vi "Packet1+Packet2Tx.vi"() -> ()   [LabVIEW 2012]
uses:
  <vilib>/addons/Modulation/Digital/General/MT Generate PSK System Parameters(M).vi
  <instrlib>/niUSRP/niUSRP Write Tx Data (CDB Cluster).vi
  <vilib>/addons/Modulation/niDMT.lvlib
panel:
  in  "Stop the \nTransmission":bool
  out "millisecond timer value 3":u32
  out "Numeric":u32
  out "output cluster":T1
  in  "Referance Cluster":T1={"Tx IQ Sampling\nRate [s/sec]"=500000.0, "Tx Frequency [Hz]"=2500000000.0, "Tx Gain [dB]"=0.0, "Tx Antenna"="TX1"} {"Tx Gain [dB]" format="%#.6p"; "Tx Frequency [Hz]" format="%#.6p"; "Tx IQ Sampling\nRate [s/sec]" format="%#.6p"}
  out "?":dbl
  out "M-PSK (4)":i32
  out "Transmission\n       Stop":bool
  in  "end of data?":bool
  out "Constellation Graph 2":T2(graph) caption="Constellation Graph"
  in  "autoscale 2":bool caption="autoscale"
  out "error out 3":errorcluster
  in  "Tab Control 2":T3(tab)
  in  "Enter Information":string
  in  "Packet Parameters 2":T4={"Guard Bits "=30, "Sync Bits"=20, "Message Bits"=128}
  in  "Packet Pad \n[samples] 2":i32=200
  in  "Blank Frame \n[samples] 2":i32=500
  out "Number of Packets in Message 2":i32=46
  in  "PN sequence order\nfor Sync Bits 2":i32=31 caption="PN sequence order (9)"
  in  "Packet Repeat 2":i32=2
  in  "Pulse Shaping Filter Parameters 2":T5={"Alpha"=0.5, "Filter Length"=6, "TX Filter"=enum."Root Raised Cos"} caption="Pulse Shaping Filter" {"Alpha" format="%.2f"}
  out "Actual Tx Parameters 2":T1={"Tx IQ Sampling\nRate [s/sec]"=200000.0, "Tx Frequency [Hz]"=2500000000.0, "Tx Gain [dB]"=0.0, "Tx Antenna"="TX1"} {"Tx Gain [dB]" format="%#.6p"; "Tx Frequency [Hz]" format="%#.6p"; "Tx IQ Sampling\nRate [s/sec]" format="%#.6p"}
  out "error out 2":errorcluster
  in  "Queue Length 2":i32=10
  in  "BPSK System Parameters 9":T6={"Samples per Symbol"=8, "symbol map"=[], "Differential PSK"=enum."disable", "PSK type"=0} caption="BPSK System Parameters" {"PSK type" items=["normal", "shifted", "offset"]; "symbol map" format="%.3f"}
  in  "BPSK System Parameters 8":T6={"Samples per Symbol"=8, "symbol map"=[], "Differential PSK"=enum."disable", "PSK type"=0} caption="BPSK System Parameters" {"PSK type" items=["normal", "shifted", "offset"]; "symbol map" format="%.3f"}
  in  "BPSK System Parameters 7":T6={"Samples per Symbol"=8, "symbol map"=[], "Differential PSK"=enum."disable", "PSK type"=0} caption="BPSK System Parameters" {"PSK type" items=["normal", "shifted", "offset"]; "symbol map" format="%.3f"}
  in  "BPSK System Parameters 6":T6={"Samples per Symbol"=8, "symbol map"=[], "Differential PSK"=enum."disable", "PSK type"=0} caption="BPSK System Parameters" {"PSK type" items=["normal", "shifted", "offset"]; "symbol map" format="%.3f"}
  in  "BPSK System Parameters 5":T6={"Samples per Symbol"=8, "symbol map"=[], "Differential PSK"=enum."disable", "PSK type"=0} caption="BPSK System Parameters" {"PSK type" items=["normal", "shifted", "offset"]; "symbol map" format="%.3f"}
  in  "BPSK System Parameters 4":T6={"Samples per Symbol"=8, "symbol map"=[], "Differential PSK"=enum."disable", "PSK type"=0} caption="BPSK System Parameters" {"PSK type" items=["normal", "shifted", "offset"]; "symbol map" format="%.3f"}
  in  "BPSK System Parameters 3":T6={"Samples per Symbol"=8, "symbol map"=[], "Differential PSK"=enum."disable", "PSK type"=0} caption="BPSK System Parameters" {"PSK type" items=["normal", "shifted", "offset"]; "symbol map" format="%.3f"}
  out "Symbol Rate\n[symbols/sec] 2":dbl=25000.0 format="%#.6p"
  out "millisecond timer value":u32
  in  "Stop after \nControl Signal Reached":bool
  in  "Tab Control":T3(tab)
  in  "Enter Control Signal\n1,2 or 3":string="Two roads diverged in a yellow wood,\nAnd sorry I could not travel both\nAnd be one traveler, long I stood\nAnd looked down one as far as I could\nTo where it bent in the undergrowth.\n\nThen took the other, as just as fair,\nAnd having perhaps the better claim,\nBecause it was grassy and wanted wear;\nThough as for that the passing there\nHad worn them really about the same.\n\nAnd both that morning equally lay\nIn leaves no step had trodden black.\nOh, I kept the first for another day!\nYet knowing how way leads on to way,\nI doubted if I should ever come back.\n\nI shall be telling this with a sigh\nSomewhere ages and ages hence:\nTwo roads diverged in a wood, and I--\nI took the one less traveled by,\nAnd that has made all the difference.\n"
  in  "Packet Parameters":T4={"Guard Bits "=30, "Sync Bits"=20, "Message Bits"=128}
  in  "Packet Pad \n[samples]":i32=200
  in  "Blank Frame \n[samples]":i32=500
  out "Number of Packets in Message":i32=46
  in  "PN sequence order\nfor Sync Bits":i32=31 caption="PN sequence order (9)"
  in  "Packet Repeat":i32=2
  in  "Select PSK Modulation Format":T7(tab)=enum."QPSK" caption="PSK"
  in  "BPSK System Parameters":T6={"Samples per Symbol"=8, "symbol map"=[], "Differential PSK"=enum."disable", "PSK type"=0} {"PSK type" items=["normal", "shifted", "offset"]; "symbol map" format="%.3f"}
  in  "QPSK System Parameters":T6={"Samples per Symbol"=8, "symbol map"=[], "Differential PSK"=enum."disable", "PSK type"=0} {"PSK type" items=["normal", "shifted", "offset"]; "symbol map" format="%.3f"}
  in  "pi/4 DQPSK System Parameters":T6={"Samples per Symbol"=8, "symbol map"=[], "Differential PSK"=enum."enable", "PSK type"=1} {"PSK type" items=["normal", "shifted", "offset"]; "symbol map" format="%.3f"}
  in  "OQPSK System Parameters":T6={"Samples per Symbol"=8, "symbol map"=[], "Differential PSK"=enum."disable", "PSK type"=2} {"PSK type" items=["normal", "shifted", "offset"]; "symbol map" format="%.3f"}
  in  "8-PSK System Parameters":T6={"Samples per Symbol"=8, "symbol map"=[], "Differential PSK"=enum."disable", "PSK type"=0} {"PSK type" items=["normal", "shifted", "offset"]; "symbol map" format="%.3f"}
  in  "16-PSK System Parameters":T6={"Samples per Symbol"=8, "symbol map"=[], "Differential PSK"=enum."disable", "PSK type"=0} {"PSK type" items=["normal", "shifted", "offset"]; "symbol map" format="%.3f"}
  in  "M":i32=4 min=2 step=2
  in  "Custom System Parameters":T6={"Samples per Symbol"=8, "symbol map"=[], "Differential PSK"=enum."disable", "PSK type"=0} {"PSK type" items=["normal", "shifted", "offset"]; "symbol map" format="%.3f"}
  in  "Pulse Shaping Filter Parameters":T5={"Alpha"=0.5, "Filter Length"=6, "TX Filter"=enum."Root Raised Cos"} caption="Pulse Shaping Filter" {"Alpha" format="%.2f"}
  in  "Tx Parameters":T1={"Tx IQ Sampling\nRate [s/sec]"=500000.0, "Tx Frequency [Hz]"=2500000000.0, "Tx Gain [dB]"=0.0, "Tx Antenna"="TX1"} {"Tx Gain [dB]" format="%#.6p"; "Tx Frequency [Hz]" format="%#.6p"; "Tx IQ Sampling\nRate [s/sec]" format="%#.6p"}
  out "Actual Tx Parameters":T1={"Tx IQ Sampling\nRate [s/sec]"=200000.0, "Tx Frequency [Hz]"=2500000000.0, "Tx Gain [dB]"=0.0, "Tx Antenna"="TX1"} {"Tx Gain [dB]" format="%#.6p"; "Tx Frequency [Hz]" format="%#.6p"; "Tx IQ Sampling\nRate [s/sec]" format="%#.6p"}
  in  "USRP IP address":refnum<k15>="192.168.10.2"
  out "error out":errorcluster
  in  "Queue Length":i32=10
  out "Constellation Graph":T2(graph)
  in  "autoscale":bool
  out "Symbol Rate\n[symbols/sec]":dbl=25000.0 format="%#.6p"
  in  "stop":bool
  # "Guard\nBand"
  # "Sync\nSeq"
  # "Packet\nNumber"
  # "Pad\nData"
  # "Blank\nFrame"
  # "Data"
  # "Guard\nBand"
  # "Sync\nSeq"
  # "Packet\nNumber"
  # "Pad\nData"
  # "Blank\nFrame"
  # "Data"
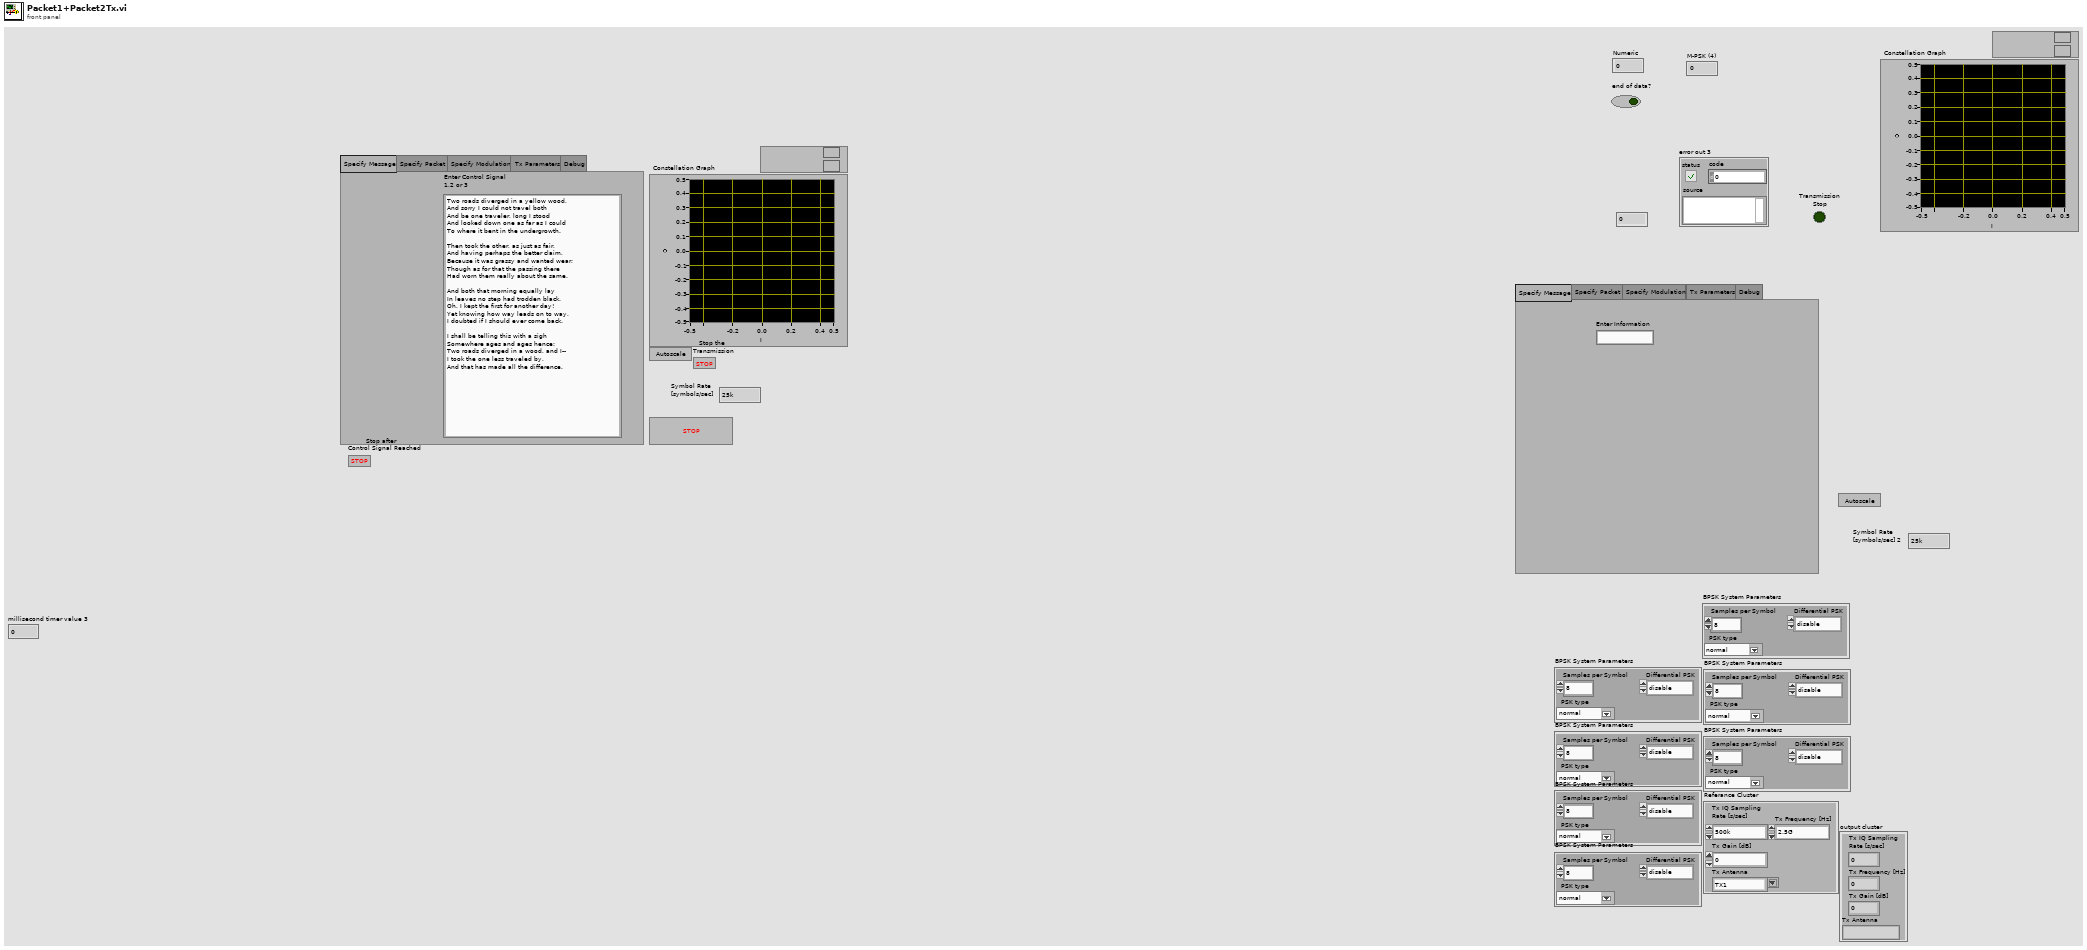
[diagram p1: front panel]
types:
  T1 = cluster{"Tx IQ Sampling\nRate [s/sec]":dbl, "Tx Frequency [Hz]":dbl, "Tx Gain [dB]":dbl, "Tx Antenna":string}
  T2 = cluster{"Decimated Array":dbl[], "Decimated Array":dbl[]}[]
  T3 = enum32{"Specify Message", "Specify Packet", "Specify Modulation", "Tx Parameters", "Debug"}
  T4 = cluster{"Guard Bits ":i32, "Sync Bits":i32, "Message Bits":i32}
  T5 = cluster{"Alpha":dbl, "Filter Length":i32, "TX Filter":enum16{"none", "Raised Cosine", "Root Raised Cos", "Gaussian"}}
  T6 = cluster{"Samples per Symbol":i32, "symbol map":cdb[], "Differential PSK":enum16{"disable", "enable"}, "PSK type":u16}
  T7 = enum32{"BPSK", "QPSK", "pi/4DQPSK", "OQPSK", "8-PSK", "16-PSK", "Custom"}
  T8 = cluster{"samples per symbol (16)":i32, "symbol map":cdb[], "differential PSK":enum16{"disable", "enable"}, "PSK type":u16}
  T9 = cluster{"s? t:f":cluster{"t0":dbl, "dt":dbl, "Y":cdb[]}, i32}
  T10 = cluster{"output complex waveform":cluster{"t0":dbl, "dt":dbl, "Y":cdb[]}, i32}
  T11 = cluster{"constellation":dbl[], "oversampled data":dbl[]}[]
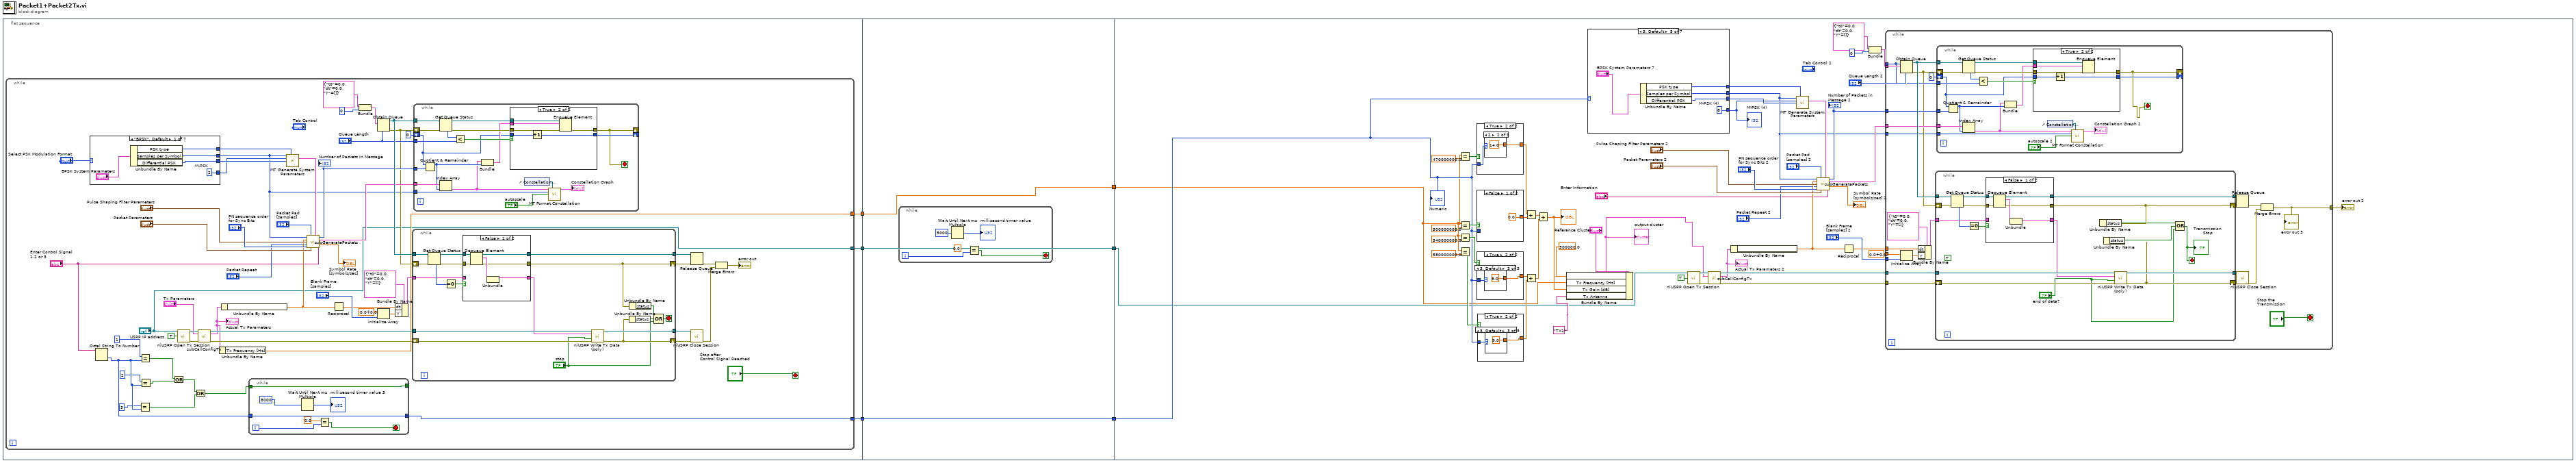
[diagram p0: block diagram]
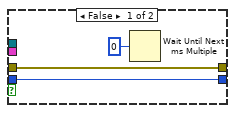
[diagram p2: hidden frame]
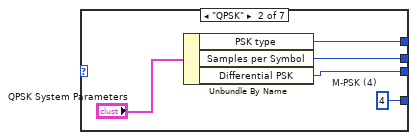
[diagram p3: hidden frame]
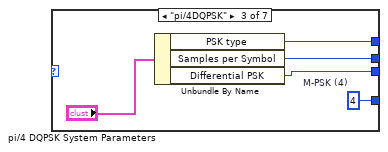
[diagram p4: hidden frame]
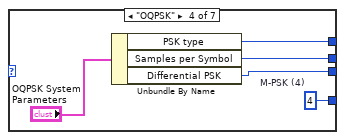
[diagram p5: hidden frame]
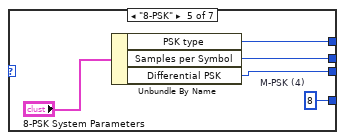
[diagram p6: hidden frame]
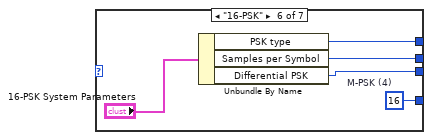
[diagram p7: hidden frame]
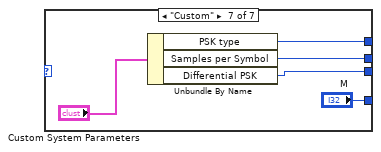
[diagram p8: hidden frame]
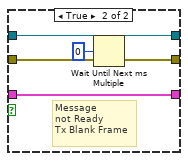
[diagram p9: hidden frame]
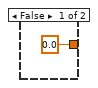
[diagram p10: hidden frame]
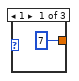
[diagram p11: hidden frame]
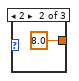
[diagram p12: hidden frame]
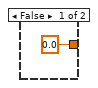
[diagram p13: hidden frame]
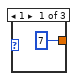
[diagram p14: hidden frame]
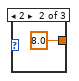
[diagram p15: hidden frame]
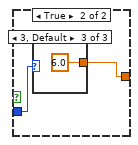
[diagram p16: hidden frame]
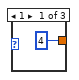
[diagram p17: hidden frame]
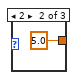
[diagram p18: hidden frame]
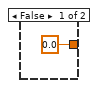
[diagram p19: hidden frame]
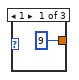
[diagram p20: hidden frame]
diagram:
  n1 = flat-sequence {
    tunnel: [w9] -> w5
    tunnel: [w8] -> w3
    tunnel: [w7] -> w1
    tunnel: [w166] -> w6
    tunnel: w5 -> [w166]
    tunnel: [w165] -> w4
    tunnel: w3 -> [w165]
    tunnel: [w164] -> w2
    tunnel: w1 -> [w164]
    tunnel: w6 -> [w174]
    tunnel: w4 -> [w173]
    tunnel: w2 -> [w172]
    frame #0 {
      n2 = while {
        tunnel: [w13] -> w9
        tunnel: [w11] -> w8
        tunnel: ["USRP IP address"] -> w7
        stop <- "Stop after \nControl Signal Reached" stop-if-true
        n3 = case shown="\"BPSK\", Default" "Select PSK Modulation Format" {
          tunnel: [w102 w106 w114 w119 w124 w130 w133] -> w27
          tunnel: [w103 w108 w113 w118 w123 w129 w134] -> w64
          tunnel: [w105 w110 w115 w120 w122 w128 "M"] -> w46
          tunnel: [w104 w109 w112 w117 w125 w127 w135] -> w35
          frame "BPSK", Default {
            w105 = 2  # M-PSK
            n4 = Unbundle By Name("BPSK System Parameters") -> ("PSK type"=w104:u16, "Samples per Symbol"=w102:i32, "Differential PSK"=w103:enum16{"disable", "enable"})
          }
          frame "QPSK" {
            w110 = 4  # M-PSK (4)
            n5 = Unbundle By Name("QPSK System Parameters") -> ("PSK type"=w109:u16, "Samples per Symbol"=w106:i32, "Differential PSK"=w108:enum16{"disable", "enable"})
          }
          frame "pi/4DQPSK" {
            w115 = 4  # M-PSK (4)
            n6 = Unbundle By Name("pi/4 DQPSK System Parameters") -> ("PSK type"=w112:u16, "Samples per Symbol"=w114:i32, "Differential PSK"=w113:enum16{"disable", "enable"})
          }
          frame "OQPSK" {
            w120 = 4  # M-PSK (4)
            n7 = Unbundle By Name("OQPSK System Parameters") -> ("PSK type"=w117:u16, "Samples per Symbol"=w119:i32, "Differential PSK"=w118:enum16{"disable", "enable"})
          }
          frame "8-PSK" {
            w122 = 8  # M-PSK (4)
            n8 = Unbundle By Name("8-PSK System Parameters") -> ("PSK type"=w125:u16, "Samples per Symbol"=w124:i32, "Differential PSK"=w123:enum16{"disable", "enable"})
          }
          frame "16-PSK" {
            w128 = 16  # M-PSK (4)
            n9 = Unbundle By Name("16-PSK System Parameters") -> ("PSK type"=w127:u16, "Samples per Symbol"=w130:i32, "Differential PSK"=w129:enum16{"disable", "enable"})
          }
          frame "Custom" {
            n10 = Unbundle By Name("Custom System Parameters") -> ("PSK type"=w135:u16, "Samples per Symbol"=w133:i32, "Differential PSK"=w134:enum16{"disable", "enable"})
          }
        }
        n11 = Octal String To Number(4:"Enter Control Signal\n1,2 or 3") -> (0:w18:u32)  [unwired: 2 in, 1 out]
        n12 = Equal?(x=3, y=w18) -> (x = y?=w20:bool)
        n13 = Equal?(x=1, y=w18) -> (x = y?=w23:bool)
        n14 = Equal?(x=2, y=w18) -> (x = y?=w22:bool)
        n15 = Or(x=w23, y=w22) -> (x .or. y?=w21:bool)
        n16 = call <instrlib>:"niUSRP Open Tx Session.vi"("device names"="USRP IP address", "reset"=TRUE) -> ("session handle out"=w38:refnum<k15>, "error out"=w37:errorcluster)  [unwired: 12 in]
        n17 = Or(x=w21, y=w20) -> (x .or. y?=w19:bool)
        n18 = call "subCallConfigTx.vi"("session handle"=w38, "Tx Parameters"="Tx Parameters", "error in"=w37) -> ("session handle out"=w45:refnum<k15>, "Actual Tx Parameters"=w12:T1, "error out"=w50:errorcluster)  [unwired: 10 in]
        "Actual Tx Parameters" <- w12
        n19 = Unbundle By Name(w12) -> ("Tx Frequency [Hz]"=w11:dbl)
        n20 = Unbundle By Name(w12) -> ("Tx IQ Sampling\nRate [s/sec]"=w28:dbl)
        n21 = while {
          tunnel: w19 -> [w71]
          tunnel: [w71] -> _
          tunnel: w18 -> [w70]
          tunnel: [w70] -> w13
          i -> [w68]
          stop <- w67 stop-if-true
          n22 = Wait Until Next ms Multiple(millisecond multiple=u32 8000) -> (millisecond timer value=→"millisecond timer value 3":u32)
          n23 = Equal?(x=0.0, y=w68) -> (x = y?=w67:bool)
        }
        n24 = call-poly <vilib>:"MT Generate System Parameters.vi"("samples per symbol (16)"=w27, "PSK type"=w35, "M-PSK (4)"=w46, "differential PSK"=w64) -> ("PSK system parameters"=w36:T8)  [unwired: 9 in, 2 out]
        n25 = call "subGeneratePackets.vi"("Samples per Symbol"=w27, "Packet Pad \n[samples]"="Packet Pad \n[samples]", "PSK system parameters"=w36, "Tx IQ Sampling\nRate [s/sec]"=w28, "Pulse Shaping Filter Parameters"="Pulse Shaping Filter Parameters", "Packet Repeat"="Packet Repeat", "PN sequence order\nfor Sync Bits"="PN sequence order\nfor Sync Bits", "Packet Parameters"="Packet Parameters", "Message Text"="Enter Control Signal\n1,2 or 3") -> ("Number of Packets"=w44:i32, "Packets"=w52:cluster{"t0":dbl, "dt":dbl, "Y":cdb[]}[], "Symbol Rate"=→"Symbol Rate\n[symbols/sec]":dbl)  [unwired: 4 in]
        "Number of Packets in Message" <- w44
        n26 = Reciprocal(x=w28) -> (1/x=w47:dbl)
        n27 = Bundle("s? t:f"=cluster{"t0":dbl, "dt":dbl, "Y":cdb[]} {"t0"=0.0, "dt"=0.0, "Y"=[]}, 0) -> (w55:T9)  [unwired: 1 in]
        n28 = Obtain Queue(max queue size (-1, unlimited)="Queue Length", element data type=w55) -> (queue out=w61:refnum<queue>, error out=w40:errorcluster)  [unwired: 3 in, 1 out]
        n29 = Initialize Array(cdb 0.0+0.0i ("element"), "Blank Frame \n[samples]") -> (w60:cdb[])
        n30 = Bundle By Name(cluster=cluster{"t0":dbl, "dt":dbl, "Y":cdb[]} {"t0"=0.0, "dt"=0.0, "Y"=[]} ("s? t:f"), "dt"=w47, "Y"=w60) -> (w59:cluster{"t0":dbl, "dt":dbl, "Y":cdb[]})
        n31 = while {
          tunnel: w45 -> [w144]
          shift-right: [w141] -> w49
          shift-left: w50 -> [w145]
          tunnel: w61 -> [w153]
          tunnel: w59 -> [w150]
          tunnel: [w149] -> w58
          tunnel: [w143] -> w48
          shift-right: [w138] -> w57
          shift-left: w40 -> [w146]
          stop <- w140 stop-if-true
          n32 = Get Queue Status(queue=w153, error in (no error)=w146) -> (queue out=w148:refnum<queue>, error out=w147:errorcluster, # elements in queue=w152:i32)  [unwired: 1 in, 5 out]
          n33 = Equal To 0?(x=w152) -> (x = 0?=w151:bool)
          n34 = case shown="False" w151 {
            tunnel: w150 -> [_ w163]
            tunnel: [w155 w163] -> w136
            tunnel: [w159 w161] -> w149
            tunnel: [w154 w162] -> w138
            tunnel: w148 -> [w158 w161]
            tunnel: w147 -> [w157 w162]
            frame False {
              n35 = Dequeue Element(queue=w158, error in (no error)=w157) -> (queue out=w159:refnum<queue>, element=w156:T9, error out=w154:errorcluster)  [unwired: 1 in, 1 out]
              n36 = Unbundle(w156) -> ("s? t:f"=w155:cluster{"t0":dbl, "dt":dbl, "Y":cdb[]})  [unwired: 1 out]
            }
            frame True {
              # "Message\nnot Ready\nTx Blank Frame"
              n37 = Wait Until Next ms Multiple(millisecond multiple=u32 0) -> ()  [unwired: 1 out]
            }
          }
          n38 = call-poly <instrlib>:"niUSRP Write Tx Data (poly).vi"("session handle"=w144, "data"=w136, "end of data?"="stop", "error in (no error)"=w145) -> ("session handle out"=w143:refnum<k15>, "error out"=w141:errorcluster)  [unwired: 10 in]
          n39 = Unbundle By Name(w141) -> ("status"=w142:bool)
          n40 = Unbundle By Name(w138) -> ("status"=w137:bool)
          n41 = Compound Arithmetic op=OR(w137, w142, "stop") -> (w140:bool)
        }
        n42 = while {
          tunnel: w61 -> [w91]
          shift-right: [w84] -> _
          shift-left: 0 -> [w80]
          tunnel: w52 -> [w81]
          tunnel: "Queue Length" -> [w83]
          tunnel: w44 -> [w82]
          shift-right: [w78] -> _
          shift-left: w40 -> [w86]
          tunnel: w27 -> [w75]
          stop <- w78 stop-if-true
          n43 = Quotient & Remainder(x=w80, y=w82) -> (x-y*floor(x/y)=w79:i32)  [unwired: 1 out]
          n44 = Index Array(array=w81, index=w79) -> (element=w73:cluster{"t0":dbl, "dt":dbl, "Y":cdb[]})
          n45 = Get Queue Status(queue=w91, error in (no error)=w86) -> (queue out=w90:refnum<queue>, error out=w87:errorcluster, # elements in queue=w89:i32)  [unwired: 1 in, 5 out]
          n46 = Less?(x=w89, y=w83) -> (x < y?=w88:bool)
          n47 = Bundle("output complex waveform"=w73, w79) -> (w85:T10)  [unwired: 1 in]
          n48 = case shown="True" w88 {
            tunnel: w87 -> [w92 w100]
            tunnel: w90 -> [_ w99]
            tunnel: [w92 w98] -> w78
            tunnel: w85 -> [_ w97]
            tunnel: w80 -> [w94 w96]
            tunnel: [w94 w95] -> w84
            frame False {
              n49 = Wait Until Next ms Multiple(millisecond multiple=u32 0) -> ()  [unwired: 1 out]
            }
            frame True {
              n50 = Increment(x=w96) -> (x+1=w95:i32)
              n51 = Enqueue Element(queue=w99, element=w97, error in (no error)=w100) -> (error out=w98:errorcluster)  [unwired: 1 in, 2 out]
            }
          }
          n52 = control-ref of="Constellation Graph"() -> (w76:refnum<vi>)
          n53 = call <vilib>:"MT Format Constellation.vi"("waveform"=w73, "constellation reference"=w76, "samples per symbol"=w75, "autoscale"="autoscale") -> ("constellation graph"=→"Constellation Graph":T11)  [unwired: 1 in, 10 out]
        }
        n54 = Release Queue(queue=w58, error in (no error)=w57) -> (error out=w34:errorcluster)  [unwired: 3 out]
        n55 = call <instrlib>:"niUSRP Close Session.vi"("session handle"=w48, "error in (no error)"=w49) -> ("error out"=w33:errorcluster)  [unwired: 13 in]
        n56 = Merge Errors(w34, w33) -> (→"error out":errorcluster)
      }
    }
    frame #1 {
      n57 = while {
        i -> [w169]
        stop <- w168 stop-if-true
        n58 = Wait Until Next ms Multiple(millisecond multiple=u32 5000) -> (millisecond timer value=→"millisecond timer value":u32)
        n59 = Equal?(x=0.0, y=w169) -> (x = y?=w168:bool)
      }
    }
    frame #2 {
      n60 = Equal?(x=w173, y=470000000.0) -> (x = y?=w182:bool)
      n61 = Equal?(x=w173, y=500000000.0) -> (x = y?=w183:bool)
      n62 = Equal?(x=w173, y=540000000.0) -> (x = y?=w184:bool)
      n63 = Equal?(x=w173, y=580000000.0) -> (x = y?=w176:bool)
      n64 = case shown="True" w182 {
        tunnel: [0.0 w242] -> w191
        tunnel: w174 -> [_ w243]
        frame False {
        }
        frame True {
          n65 = case shown="2" w243 {
            tunnel: [9 14.0 18.0] -> w242
            frame 1 {
            }
            frame 2 {
            }
            frame 3, Default {
            }
          }
        }
      }
      n66 = case shown="False" w183 {
        tunnel: [0.0 w236] -> w190
        tunnel: w174 -> [_ w237]
        frame False {
        }
        frame True {
          n67 = case shown="3, Default" w237 {
            tunnel: [4 5.0 6.0] -> w236
            frame 1 {
            }
            frame 2 {
            }
            frame 3, Default {
            }
          }
        }
      }
      n68 = case shown="True" w184 {
        tunnel: [0.0 w230] -> w189
        tunnel: w174 -> [_ w231]
        frame False {
        }
        frame True {
          n69 = case shown="3, Default" w231 {
            tunnel: [7 8.0 9.0] -> w230
            frame 1 {
            }
            frame 2 {
            }
            frame 3, Default {
            }
          }
        }
      }
      n70 = case shown="True" w176 {
        tunnel: [0.0 w224] -> w175
        tunnel: w174 -> [_ w225]
        frame False {
        }
        frame True {
          n71 = case shown="3, Default" w225 {
            tunnel: [7 8.0 9.0] -> w224
            frame 1 {
            }
            frame 2 {
            }
            frame 3, Default {
            }
          }
        }
      }
      n72 = Add(x=w191, y=w190) -> (x+y=w193:dbl)
      n73 = Add(x=w189, y=w175) -> (x+y=w192:dbl)
      n74 = Add(x=w193, y=w192) -> (x+y=w180:dbl)
      "?" <- w180
      n75 = Bundle By Name(cluster="Referance Cluster", "Tx IQ Sampling\nRate [s/sec]"=500000.0, "Tx Frequency [Hz]"=w173, "Tx Gain [dB]"=w180, "Tx Antenna"="TX1") -> (w178:T1)
      "output cluster" <- w178
      n76 = case shown="3, Default" w174 {
        tunnel: [w328 w333 w340 w345 w350 w356 w359] -> w197
        tunnel: [w329 w334 w339 w344 w349 w355 w360] -> w222
        tunnel: [w331 w336 w341 w346 w348 w354 0 ("M-PSK (4)")] -> w213
        tunnel: [w330 w335 w338 w343 w351 w353 w361] -> w203
        frame 1 {
          w331 = 2  # M-PSK
          n77 = Unbundle By Name("BPSK System Parameters 3") -> ("PSK type"=w330:u16, "Samples per Symbol"=w328:i32, "Differential PSK"=w329:enum16{"disable", "enable"})
        }
        frame 2 {
          w336 = 4  # M-PSK (4)
          n78 = Unbundle By Name("BPSK System Parameters 4") -> ("PSK type"=w335:u16, "Samples per Symbol"=w333:i32, "Differential PSK"=w334:enum16{"disable", "enable"})
        }
        frame 4 {
          w341 = 4  # M-PSK (4)
          n79 = Unbundle By Name("BPSK System Parameters 5") -> ("PSK type"=w338:u16, "Samples per Symbol"=w340:i32, "Differential PSK"=w339:enum16{"disable", "enable"})
        }
        frame 5 {
          w346 = 4  # M-PSK (4)
          n80 = Unbundle By Name("BPSK System Parameters 6") -> ("PSK type"=w343:u16, "Samples per Symbol"=w345:i32, "Differential PSK"=w344:enum16{"disable", "enable"})
        }
        frame 3, Default {
          w348 = 8  # M-PSK (4)
          n81 = Unbundle By Name("BPSK System Parameters 7") -> ("PSK type"=w351:u16, "Samples per Symbol"=w350:i32, "Differential PSK"=w349:enum16{"disable", "enable"})
        }
        frame 6 {
          w354 = 16  # M-PSK (4)
          n82 = Unbundle By Name("BPSK System Parameters 8") -> ("PSK type"=w353:u16, "Samples per Symbol"=w356:i32, "Differential PSK"=w355:enum16{"disable", "enable"})
        }
        frame 7 {
          n83 = Unbundle By Name("BPSK System Parameters 9") -> ("PSK type"=w361:u16, "Samples per Symbol"=w359:i32, "Differential PSK"=w360:enum16{"disable", "enable"})
        }
      }
      "M-PSK (4)" <- w213
      n84 = call <instrlib>:"niUSRP Open Tx Session.vi"("device names"=w172, "reset"=TRUE) -> ("session handle out"=w206:refnum<k15>, "error out"=w205:errorcluster)  [unwired: 12 in]
      n85 = call "subCallConfigTx.vi"("session handle"=w206, "Tx Parameters"=w178, "error in"=w205) -> ("session handle out"=w212:refnum<k15>, "Actual Tx Parameters"=w211:T1, "error out"=w215:errorcluster)  [unwired: 10 in]
      "Actual Tx Parameters 2" <- w211
      n86 = Unbundle By Name(w211) -> ("Tx IQ Sampling\nRate [s/sec]"=w198:dbl)
      n87 = call-poly <vilib>:"MT Generate System Parameters.vi"("samples per symbol (16)"=w197, "PSK type"=w203, "M-PSK (4)"=w213, "differential PSK"=w222) -> ("PSK system parameters"=w204:T8)  [unwired: 9 in, 2 out]
      n88 = call "subGeneratePackets.vi"("Samples per Symbol"=w197, "Packet Pad \n[samples]"="Packet Pad \n[samples] 2", "PSK system parameters"=w204, "Tx IQ Sampling\nRate [s/sec]"=w198, "Pulse Shaping Filter Parameters"="Pulse Shaping Filter Parameters 2", "Packet Repeat"="Packet Repeat 2", "PN sequence order\nfor Sync Bits"="PN sequence order\nfor Sync Bits 2", "Packet Parameters"="Packet Parameters 2", "Message Text"="Enter Information") -> ("Number of Packets"=w210:i32, "Packets"=w216:cluster{"t0":dbl, "dt":dbl, "Y":cdb[]}[], "Symbol Rate"=→"Symbol Rate\n[symbols/sec] 2":dbl)  [unwired: 4 in]
      "Number of Packets in Message 2" <- w210
      n89 = Reciprocal(x=w198) -> (1/x=w214:dbl)
      n90 = Bundle("s? t:f"=cluster{"t0":dbl, "dt":dbl, "Y":cdb[]} {"t0"=0.0, "dt"=0.0, "Y"=[]}, 0) -> (w218:T9)  [unwired: 1 in]
      n91 = while {
        tunnel: cdb 0.0+0.0i ("element") -> [w270]
        tunnel: "Blank Frame \n[samples] 2" -> [w269]
        tunnel: w218 -> [w263]
        tunnel: "Queue Length 2" -> [w261]
        tunnel: w216 -> [w260]
        tunnel: w215 -> [w259]
        tunnel: w214 -> [w256]
        tunnel: w212 -> [w255]
        tunnel: w210 -> [w254]
        tunnel: [w249] -> w202
        tunnel: w197 -> [w248]
        stop <- "Stop the \nTransmission" stop-if-true
        n92 = Obtain Queue(max queue size (-1, unlimited)=w261, element data type=w263) -> (queue out=w268:refnum<queue>, error out=w252:errorcluster)  [unwired: 3 in, 1 out]
        n93 = Initialize Array(w270, w269) -> (w267:cdb[])
        n94 = Bundle By Name(cluster=cluster{"t0":dbl, "dt":dbl, "Y":cdb[]} {"t0"=0.0, "dt"=0.0, "Y"=[]} ("s? t:f"), "dt"=w256, "Y"=w267) -> (w266:cluster{"t0":dbl, "dt":dbl, "Y":cdb[]})
        n95 = while {
          tunnel: w255 -> [w307]
          shift-right: [w304] -> w258
          shift-left: w259 -> [w308]
          tunnel: w268 -> [w316]
          tunnel: w266 -> [w313]
          tunnel: [w312] -> w265
          tunnel: [w306] -> w257
          shift-right: [w303] -> w264
          shift-left: w252 -> [w309]
          stop <- w300 stop-if-true
          (unwired) TRUE
          n96 = Get Queue Status(queue=w316, error in (no error)=w309) -> (queue out=w311:refnum<queue>, error out=w310:errorcluster, # elements in queue=w315:i32)  [unwired: 1 in, 5 out]
          n97 = Equal To 0?(x=w315) -> (x = 0?=w314:bool)
          n98 = case shown="False" w314 {
            tunnel: w313 -> [_ w326]
            tunnel: [w318 w326] -> w301
            tunnel: [w322 w324] -> w312
            tunnel: [w317 w325] -> w303
            tunnel: w311 -> [w321 w324]
            tunnel: w310 -> [w320 w325]
            frame False {
              n99 = Dequeue Element(queue=w321, error in (no error)=w320) -> (queue out=w322:refnum<queue>, element=w319:T9, error out=w317:errorcluster)  [unwired: 1 in, 1 out]
              n100 = Unbundle(w319) -> ("s? t:f"=w318:cluster{"t0":dbl, "dt":dbl, "Y":cdb[]})  [unwired: 1 out]
            }
            frame True {
              # "Message\nnot Ready\nTx Blank Frame"
              n101 = Wait Until Next ms Multiple(millisecond multiple=u32 0) -> ()  [unwired: 1 out]
            }
          }
          n102 = Unbundle By Name(w303) -> ("status"=w302:bool)
          n103 = call-poly <instrlib>:"niUSRP Write Tx Data (poly).vi"("session handle"=w307, "data"=w301, "end of data?"="end of data?", "error in (no error)"=w308) -> ("session handle out"=w306:refnum<k15>, "error out"=w304:errorcluster)  [unwired: 10 in]
          n104 = Unbundle By Name(w304) -> ("status"=w305:bool)
          n105 = Compound Arithmetic op=OR(w302, w305, "end of data?") -> (w300:bool)
          "Transmission\n       Stop" <- w300
        }
        n106 = while {
          tunnel: w268 -> [w289]
          shift-right: [w282] -> _
          shift-left: 0 -> [w278]
          tunnel: w260 -> [w279]
          tunnel: w261 -> [w281]
          tunnel: w254 -> [w280]
          shift-right: [w271] -> _
          shift-left: w252 -> [w284]
          tunnel: w248 -> [w274]
          stop <- w271 stop-if-true
          n107 = Quotient & Remainder(x=w278, y=w280) -> (x-y*floor(x/y)=w277:i32)  [unwired: 1 out]
          n108 = Index Array(array=w279, index=w277) -> (element=w272:cluster{"t0":dbl, "dt":dbl, "Y":cdb[]})
          n109 = Get Queue Status(queue=w289, error in (no error)=w284) -> (queue out=w288:refnum<queue>, error out=w285:errorcluster, # elements in queue=w287:i32)  [unwired: 1 in, 5 out]
          n110 = Less?(x=w287, y=w281) -> (x < y?=w286:bool)
          n111 = Bundle("output complex waveform"=w272, w277) -> (w283:T10)  [unwired: 1 in]
          n112 = case shown="True" w286 {
            tunnel: w285 -> [w290 w298]
            tunnel: w288 -> [_ w297]
            tunnel: [w290 w296] -> w271
            tunnel: w283 -> [_ w295]
            tunnel: w278 -> [w292 w294]
            tunnel: [w292 w293] -> w282
            frame False {
              n113 = Wait Until Next ms Multiple(millisecond multiple=u32 0) -> ()  [unwired: 1 out]
            }
            frame True {
              n114 = Increment(x=w294) -> (x+1=w293:i32)
              n115 = Enqueue Element(queue=w297, element=w295, error in (no error)=w298) -> (error out=w296:errorcluster)  [unwired: 1 in, 2 out]
            }
          }
          n116 = control-ref of="Constellation Graph 2"() -> (w275:refnum<vi>)
          n117 = call <vilib>:"MT Format Constellation.vi"("waveform"=w272, "constellation reference"=w275, "samples per symbol"=w274, "autoscale"="autoscale 2") -> ("constellation graph"=→"Constellation Graph 2":T11)  [unwired: 1 in, 10 out]
        }
        n118 = Release Queue(queue=w265, error in (no error)=w264) -> (error out=w251:errorcluster)  [unwired: 3 out]
        n119 = call <instrlib>:"niUSRP Close Session.vi"("session handle"=w257, "error in (no error)"=w258) -> ("error out"=w250:errorcluster)  [unwired: 13 in]
        n120 = Merge Errors(w251, w250) -> (w249:errorcluster)
        "error out 3" <- w249
      }
      "error out 2" <- w202
      "Numeric" <- w174
    }
  }
